vi "File Creator.vi"(8 "prompt":string, 9 "Amplifier Channel 1":T1 {"Amplifier Model" items=["Select a Model", "AM 1700", "BMA 200"]}, 10 "User Data Channel 1":T2, 11 "Use Channel in":bool) -> (3 "Refnum out":refnum<k34>)   [LabVIEW 2014]
panel:
  # "Blue for On\nOrange for Off"
  # "DC"
  # "AC"
  # "Blue for AC and Orange for DC"
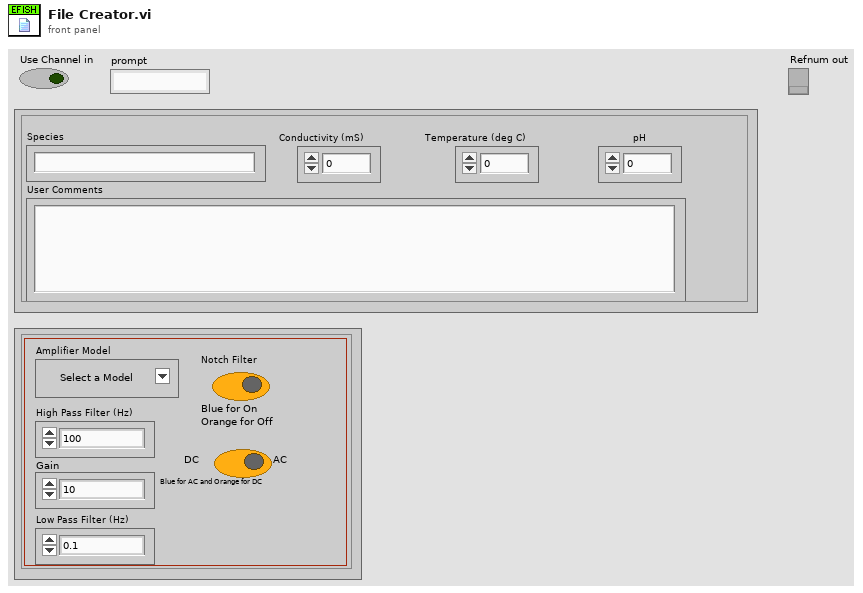
[diagram p1: front panel]
types:
  T1 = cluster{"Low Pass Filter (Hz)":enum16{"0.1", "1", "3", "10", "30", "100", "300"}, "Gain ":enum16{"10", "20", "50", "100", "200", "500", "1000", "2k", "5k", "10k", "20k", "50k"}, "High Pass Filter (Hz)":enum16{"100", "500", "1000", "3000", "5000", "10,000", "20,000", "30,000", "50,000"}, "Notch Filter":bool, "Amplifier Model":u16, "AC/DC Switch":bool}
  T2 = cluster{"pH":dbl, "Conductivity (mS)":dbl, "Temperature (deg C)":dbl, "User Comments":string, "Species":string}
  T3 = enum16{"open", "open or create", "create or replace", "create", "open (read-only)"}
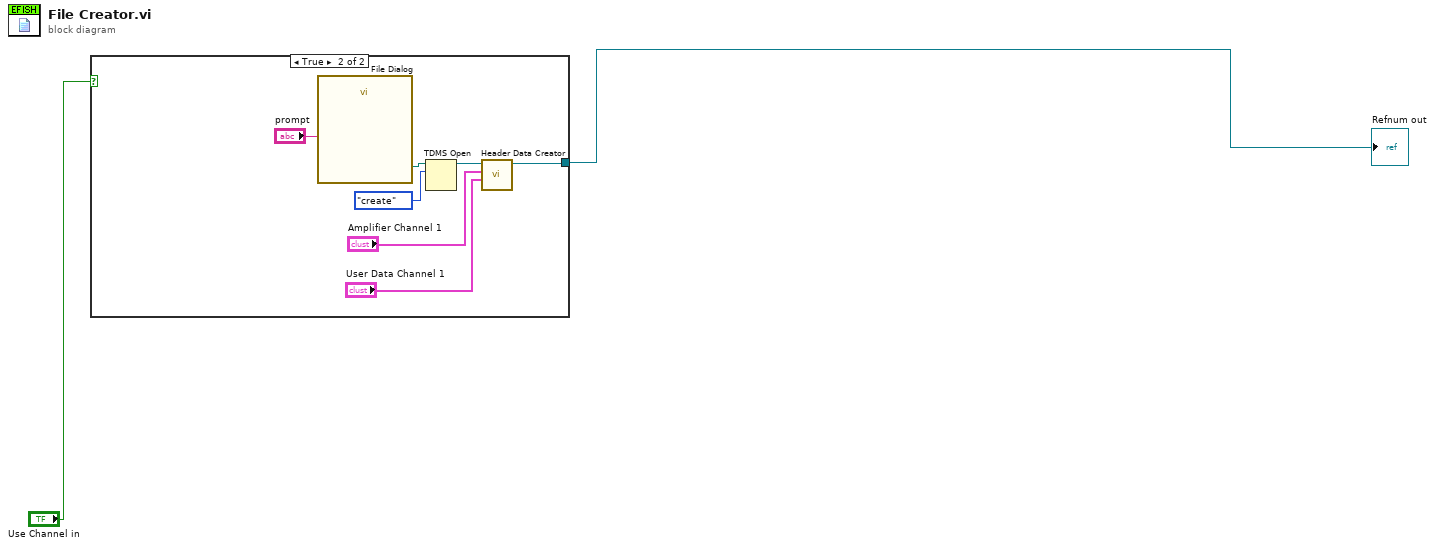
[diagram p0: block diagram]
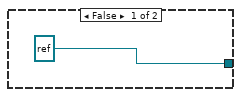
[diagram p2: hidden frame]
diagram:
  n1 = case shown="True" "Use Channel in" {
    tunnel: [refnum<k34> refnum ("tdms file out") w5] -> w1
    frame False {
    }
    frame True {
      n2 = call "File Dialog"("prompt"="prompt") -> ("selected path"=w9:path)  [unwired: 11 in, 3 out]
      n3 = TDMS Open(10:T3."create" ("operation (0:open)"), 11:w9) -> (3:w8:refnum<k34>)  [unwired: 5 in, 1 out]
      n4 = call "Header Data Creator.vi"("tdms file in"=w8, "Amplifier Metadata"="Amplifier Channel 1", "User Data"="User Data Channel 1") -> ("tdms file out"=w5:refnum<k34>)  [unwired: 6 in, 1 out]
    }
  }
  "Refnum out" <- w1
